vi "Sub_Preprocessing_Create_Accel_Datastream.vi"() -> (1 "Start time":dbl, 2 "Sample rate":dbl, 3 "Experimental Replay":T1)   [LabVIEW 2021]
panel:
  # "Generate data from file"
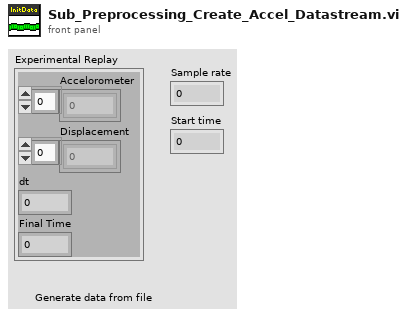
[diagram p1: front panel]
types:
  T1 = cluster{"Accelorometer":dbl[], "Displacement":dbl[], "dt":dbl, "Final Time":dbl}
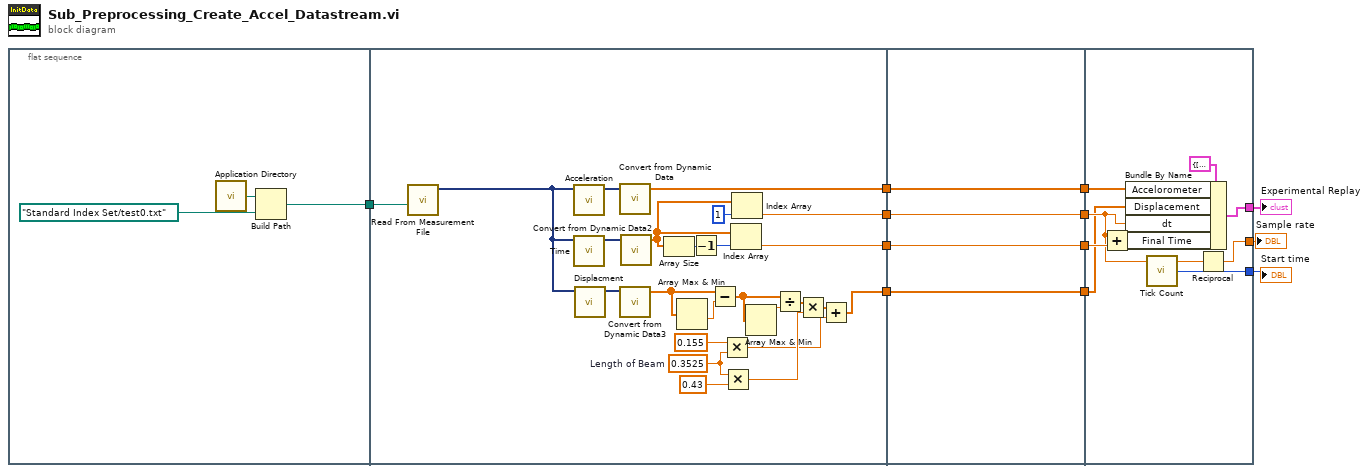
[diagram p0: block diagram]
diagram:
  n1 = flat-sequence {
    tunnel: [w13] -> w12
    tunnel: w12 -> [w39]
    tunnel: [w35] -> w8
    tunnel: [w34] -> w6
    tunnel: [w33] -> w4
    tunnel: [w20] -> w2
    tunnel: w8 -> [w43]
    tunnel: [w43] -> w7
    tunnel: w6 -> [w42]
    tunnel: [w42] -> w5
    tunnel: w4 -> [w41]
    tunnel: [w41] -> w3
    tunnel: w2 -> [w40]
    tunnel: [w40] -> w1
    tunnel: w7 -> [w52]
    tunnel: w5 -> [w45]
    tunnel: w3 -> [w47]
    tunnel: [w50] -> w9
    tunnel: [w48] -> w11
    tunnel: [w49] -> w10
    tunnel: w1 -> [w44]
    frame #0 {
      n2 = call <vilib>:"Application Directory.vi"() -> ("Application Directory"=w15:path)
      n3 = Build Path(base path=w15, name or relative path=path "Standard Index Set/test0.txt") -> (appended path=w13:path)
    }
    frame #1 {
      w26 = 0.3525  # Length of Beam
      n4 = call "Read From Measurement File"("Filename"=w39) -> ("Signals"=w29:dynamicdata)  [unwired: 5 in, 5 out]
      n5 = call "Acceleration"("Signals"=w29) -> ("Signal Out"=w38:dynamicdata)  [unwired: 9 in, 1 out]
      n6 = call "Time"("Signals"=w29) -> ("Signal Out"=w37:dynamicdata)  [unwired: 9 in, 1 out]
      n7 = call "Displacment"("Signals"=w29) -> ("Signal Out"=w28:dynamicdata)  [unwired: 9 in, 1 out]
      n8 = call "Convert from Dynamic Data"("Dynamic Data Type"=w38) -> ("Array"=w35:dbl[])  [unwired: 3 in]
      n9 = call "Convert from Dynamic Data3"("Dynamic Data Type"=w28) -> ("Array"=w19:dbl[])  [unwired: 3 in]
      n10 = call "Convert from Dynamic Data2"("Dynamic Data Type"=w37) -> ("Array"=w31:dbl[])  [unwired: 3 in]
      n11 = Array Size(array=w31) -> (size(s)=w32:i32)
      n12 = Array Max & Min(array=w19) -> (min value=w24:dbl)  [unwired: 3 out]
      n13 = Decrement(x=w32) -> (x-1=w30:i32)
      n14 = Subtract(x=w19, y=w24) -> (x-y=w18:dbl[])
      n15 = Multiply(x=0.155, y=w26) -> (x*y=w21:dbl)
      n16 = Multiply(x=w26, y=0.43) -> (x*y=w22:dbl)
      n17 = Index Array(array=w31, index=w30) -> (element=w33:dbl)
      n18 = Index Array(array=w31, index=1) -> (element=w34:dbl)
      n19 = Array Max & Min(array=w18) -> (max value=w17:dbl)  [unwired: 3 out]
      n20 = Divide(x=w18, y=w17) -> (x/y=w16:dbl[])
      n21 = Multiply(x=w16, y=w22) -> (x*y=w23:dbl[])
      n22 = Add(x=w23, y=w21) -> (x+y=w20:dbl[])
    }
    frame #2 {
    }
    frame #3 {
      n23 = Add(x=w45, y=w47) -> (x+y=w46:dbl)
      n24 = Bundle By Name(cluster=T1 {"Accelorometer"=[], "Displacement"=[], "dt"=0.0, "Final Time"=0.0} ("input cluster"), "Accelorometer"=w52, "Displacement"=w44, "dt"=w45, "Final Time"=w46) -> (w50:T1)
      n25 = call "Tick Count"() -> ("Tick Count(uSec)"=w49:u32)
      n26 = Reciprocal(x=w45) -> (1/x=w48:dbl)
    }
  }
  "Sample rate" <- w11
  "Start time" <- w10
  "Experimental Replay" <- w9
